vi "Finalize To JSON.vi"(8 "error in (no error)":errorcluster, 11 "UDP Thread Configuration in":refnum<class "UDP Thread Configuration.lvclass">) -> (0 "error out":errorcluster, 1 "format version":T1, 2 "json":string, 3 "UDP Thread Configuration out":refnum<class "UDP Thread Configuration.lvclass">)   [LabVIEW 2017, in "DSF Core.lvlib" / "UDP Thread Configuration.lvclass"]
uses:
  UDP Thread Configuration.lvclass
  Classes/Configuration/Configuration.lvclass
  C:/Git/DSF/Core/Classes/Configuration/Configuration.lvclass
  Typedefs/DSF Version Info.ctl
  DSF Core.lvlib
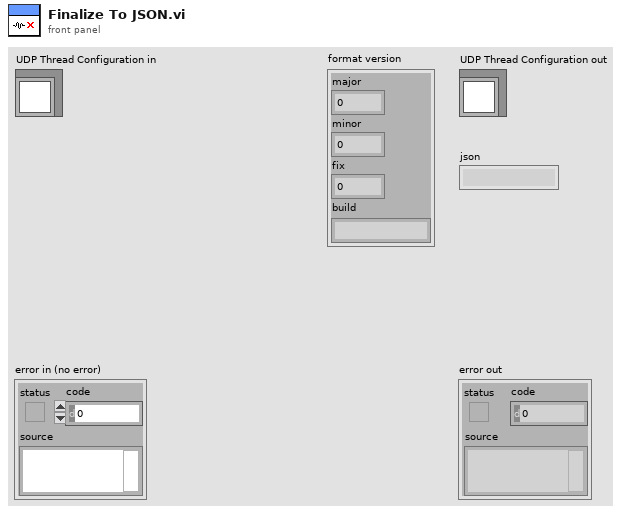
[diagram p1: front panel]
types:
  T1 = typedef "DSF Core.lvlib/DSF Version Info.ctl" = cluster{"major":i32, "minor":i32, "fix":i32, "build":string}
  T2 = typedef "DSF Core.lvlib/UDP Thread Configuration.lvclass/Thread Settings.ctl" = cluster{"local port":u16, "local address":u32}
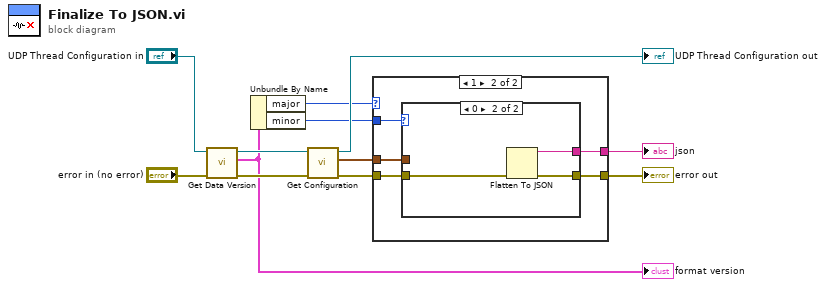
[diagram p0: block diagram]
diagram:
  n1 = call "Get Data Version.vi"("error in (no error)"="error in (no error)", "Configuration in"="UDP Thread Configuration in") -> ("error out"=w7:errorcluster, "data version"=w6:T1, "Configuration out"=w8:refnum<class "UDP Thread Configuration.lvclass">)  [unwired: 7 in]
  "format version" <- w6
  n2 = Unbundle By Name(w6) -> ("major"=w1:i32, "minor"=w2:i32)
  n3 = call "Get Configuration.vi"("error in (no error)"=w7, "DSF UDP Thread Configuration in"=w8) -> ("error out"=w5:errorcluster, "thread settings"=w4:T2, "DSF UDP Thread Configuration out"=→"UDP Thread Configuration out":refnum<class "UDP Thread Configuration.lvclass">)  [unwired: 7 in]
  n4 = case shown="1" w1 {
    tunnel: w2 -> [_ w18]
    tunnel: w5 -> [w13 w17]
    tunnel: [w13 w16] -> w10
    tunnel: [_ w15] -> w9
    tunnel: w4 -> [_ w14]
    frame 0, Default {
    }
    frame 1 {
      n5 = case shown="0" w18 {
        tunnel: w17 -> [w19 w22]
        tunnel: [w19 w21] -> w16
        tunnel: [_ w20] -> w15
        tunnel: w14 -> [_ _]
        frame -1, Default {
        }
        frame 0 {
          n6 = Flatten To JSON(error in (no error)=w22) -> (JSON string=w20:string, 11:w21:errorcluster)  [unwired: 2 in]
        }
      }
    }
  }
  "error out" <- w10
  "json" <- w9
